vi "Core Action.vi"(8 "error in (no error)":errorcluster, 10 "SECS-II Class":refnum<class "SECS-II Class.lvclass">, 11 "09-Host Requsts Individual Report in":refnum<class "09-Host Requsts Individual Report.lvclass">) -> (0 "error out":errorcluster, 2 "SECS-II Class Out":refnum<class "SECS-II Class.lvclass">, 3 "09-Host Requsts Individual Report out":refnum<class "09-Host Requsts Individual Report.lvclass">)   [LabVIEW 2020, in "SECS Scenarios.lvlib" / "09-Host Requsts Individual Report.lvclass"]
uses:
  09-Host Requsts Individual Report.lvclass
  D:/Dropbox/SECS/SECS_GEM v1.1.0/Com/SECS Scenarios/Scenarios Class/Scenarios Class.lvclass
  SECS Communication/SECS-II Class/SECS-II Class.lvclass
  SECS Communication/S6 Message Class/S6 Message Class.lvclass
  D:/Dropbox/SECS/SECS_GEM v1.1.0/Com/SECS Communication/SECS-II Class/SECS-II Class.lvclass
  Scenarios Class/Reply State.ctl
  Scenarios Class/Scenarios Class.lvclass/Scenarios Class.ctl
  Scenarios Class/Write Reply State.vi
  Scenarios Class/Read HSMS Class.vi
  SECS Communication/HSMS Class/HSMS Class.lvclass
  Scenarios Class/Scenarios Class.lvclass
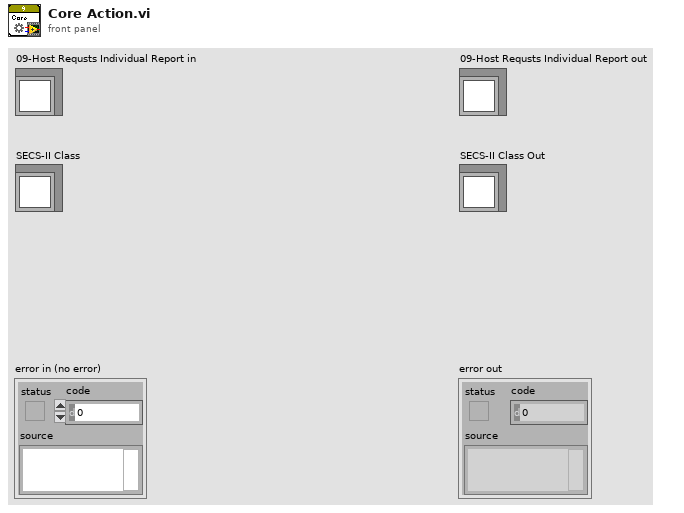
[diagram p1: front panel]
types:
  T1 = typedef "SECS Communication.lvlib/SECS-II Class.lvclass/Format Code.ctl" = enum16{"L", "A", "B", "Boolean", "J", "I1", "I2", "I4", "I8", "U1", "U2", "U4", "U8", "F4", "F8", "Char"}
  T2 = typedef "SECS Scenarios.lvlib/Scenarios Class.lvclass/Reply State.ctl" = enum16{"OK", "Illegal Data", "Unknown Stream", "Unknown Function", "Off-Line", "T3 Timeout", "Inner-Timeout"}
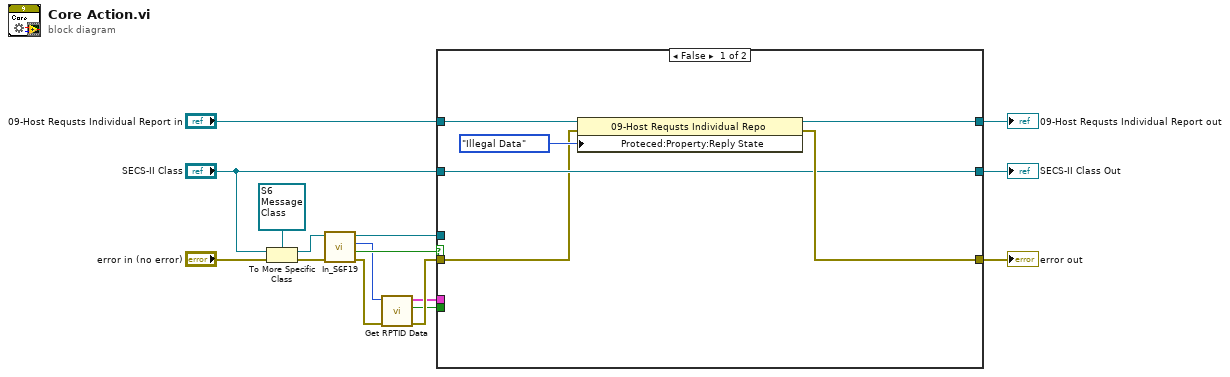
[diagram p0: block diagram]
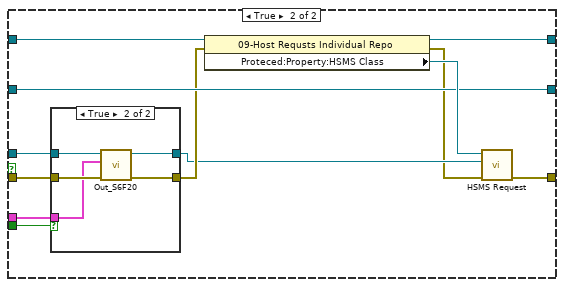
[diagram p2: hidden frame]
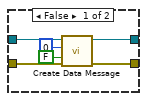
[diagram p3: hidden frame]
diagram:
  n1 = To More Specific Class(target class=refnum<class "S6 Message Class.lvclass"> refnum ("SECS Communication.lvlib:S6 Message Class.lvclass"), reference="SECS-II Class", error in="error in (no error)") -> (specific class reference=w15:refnum<class "S6 Message Class.lvclass">, error out=w16:errorcluster)
  n2 = call "In_S6F19.vi"("error in (no error)"=w16, "S6 Message Class in"=w15) -> ("error out"=w5:errorcluster, "OK?"=w6:bool, "RPTID"=w4:u32, "S6 Message Class out"=w14:refnum<class "S6 Message Class.lvclass">)  [unwired: 6 in]
  n3 = call "Get RPTID Data.vi"("error in (no error)"=w5, "RPTID"=w4) -> ("error out"=w3:errorcluster, "OK"=w1:bool, "Value"=w2:cluster{"Format Code":T1, "Value":variant}[])  [unwired: 7 in]
  n4 = case shown="False" w6 {
    tunnel: "09-Host Requsts Individual Report in" -> [w22 w34]
    tunnel: [w21 w32] -> w12
    tunnel: [w20 w31] -> w13
    tunnel: w14 -> [_ w29]
    tunnel: "SECS-II Class" -> [w18 w30]
    tunnel: [w18 w30] -> w7
    tunnel: w3 -> [w17 w28]
    tunnel: w2 -> [_ w27]
    tunnel: w1 -> [_ w26]
    frame False {
      n5 = property class="09-Host Requsts Individual Repo"(reference=w22, error in=w17, "Proteced:Property:Reply State"=Reply_State."Illegal Data" ("Reply State")) -> (reference out=w21:refnum<class "09-Host Requsts Individual Report.lvclass">, error out=w20:errorcluster)
    }
    frame True {
      n6 = case shown="True" w26 {
        tunnel: w27 -> [_ w43]
        tunnel: w29 -> [w40 w45]
        tunnel: [w39 w42] -> w24
        tunnel: [w38 w41] -> w25
        tunnel: w28 -> [w37 w44]
        frame False {
          n7 = call "Create Data Message.vi"("error in (no error)"=w37, "W-Bit"=FALSE, "Function"=u8 0, "SECS-II Class in"=w40) -> ("error out"=w38:errorcluster, "SECS-II Class out"=w39:refnum<class "S6 Message Class.lvclass">)  [unwired: 6 in]
        }
        frame True {
          n8 = call "Out_S6F20.vi"("error in (no error)"=w44, "Value"=w43, "S6 Message Class in"=w45) -> ("error out"=w41:errorcluster, "S6 Message Class out"=w42:refnum<class "S6 Message Class.lvclass">)  [unwired: 7 in]
        }
      }
      n9 = property class="09-Host Requsts Individual Repo"(reference=w34, error in=w25) -> (reference out=w32:refnum<class "09-Host Requsts Individual Report.lvclass">, error out=w23:errorcluster, "Proteced:Property:HSMS Class"=w33:refnum<class "HSMS Class.lvclass">)
      n10 = call "HSMS Request.vi"("error in (no error)"=w23, "SECS-II Class In"=w24, "HSMS Class in"=w33) -> ("error out"=w31:errorcluster)  [unwired: 7 in, 1 out]
    }
  }
  "error out" <- w13
  "09-Host Requsts Individual Report out" <- w12
  "SECS-II Class Out" <- w7
